vi "Check Instrument Serial Number.vi"(7 "Seq Count":i32, 8 "error in (no error)":errorcluster, 9 "Instrument IDN String (\"\")":string, 11 "Instrument Record":T1) -> (0 "error out":errorcluster)   [LabVIEW 2011]
uses:
  typedefs/Instrument Record.ctl
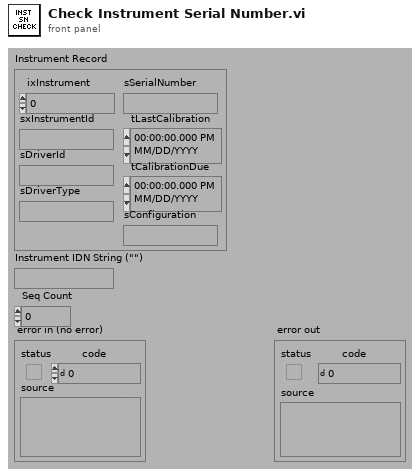
[diagram p1: front panel]
types:
  T1 = typedef "Instrument Record.ctl" = cluster{"ixInstrument":i32, "sxInstrumentId":string, "sDriverId":string, "sDriverType":string, "sSerialNumber":string, "tLastCalibration":timestamp, "tCalibrationDue":timestamp, "sConfiguration":string}
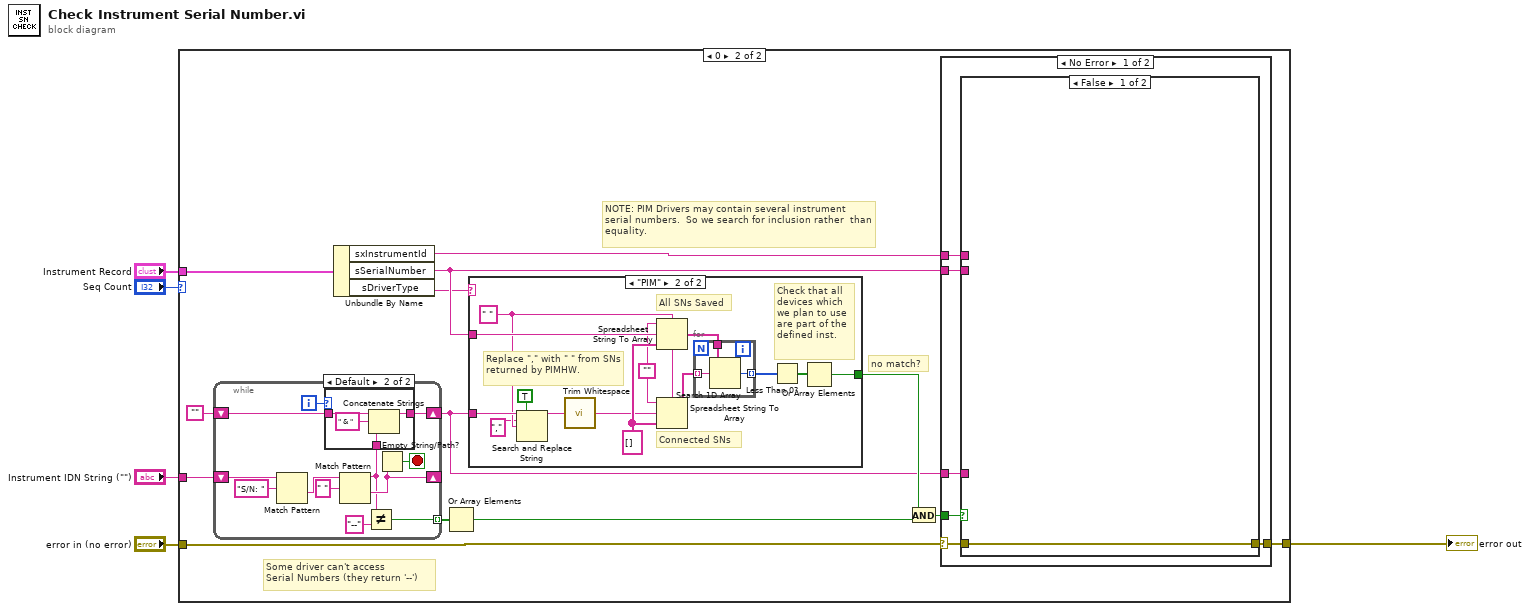
[diagram p0: block diagram]
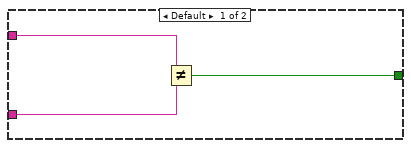
[diagram p3: hidden frame]
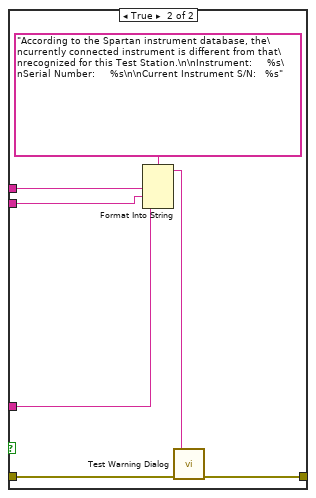
[diagram p5: hidden frame]
diagram:
  n1 = case shown="0" "Seq Count" {
    tunnel: "Instrument Record" -> [_ w18]
    tunnel: [w6 w17] -> w4
    tunnel: "error in (no error)" -> [w6 w16]
    tunnel: "Instrument IDN String (\"\")" -> [_ w13]
    frame Default {
      # "Do not run check if it is not the first time the sequence is run."
    }
    frame 0 {
      # "no match?"
      # "NOTE: PIM Drivers may contain several instrument serial numbers.  So we search for inclusion rather  than equality."
      # "Some driver can't access\nSerial Numbers (they return '--')"
      n2 = while {
        shift-right: [w45] -> _
        shift-left: w13 -> [w50]
        tunnel: [w46] -> w12 mode=indexing
        shift-right: [w41] -> w7
        shift-left: "" -> [w42]
        i -> [w43]
        stop <- w44 stop-if-true
        n3 = Match Pattern(string=w50, regular expression="S/N: ") -> (after substring=w49:string)  [unwired: 4 out]
        n4 = Match Pattern(string=w49, regular expression=" ") -> (before substring=w40:string, after substring=w45:string)  [unwired: 3 out]
        n5 = case shown="Default" w43 {
          tunnel: w42 -> [_ w56]
          tunnel: [w52 w54] -> w41
          tunnel: w40 -> [w52 w55]
          frame 0 {
          }
          frame Default {
            n6 = Concatenate Strings(w56, " & " ("string"), w55) -> (w54:string)
          }
        }
        n7 = Not Equal?(x=w40, y="--" ("x")) -> (x != y?=w46:bool)
        n8 = Empty String/Path?(string/path=w45) -> (empty?=w44:bool)
      }
      n9 = Unbundle By Name(w18) -> ("sxInstrumentId"=w19:string, "sSerialNumber"=w14:string, "sDriverType"=w8:string)
      n10 = Or Array Elements(Boolean array=w12) -> (logical OR=w9:bool)
      n11 = case shown="\"PIM\"" w8 {
        tunnel: w14 -> [w22 w35]
        tunnel: w7 -> [w21 w27]
        tunnel: [w20 w30] -> w10
        frame Default {
          n12 = Not Equal?(x=w22, y=w21) -> (x != y?=w20:bool)
        }
        frame "PIM" {
          w34 = ""
          w36 = string[] []
          w26 = " " ("delimiter (Tab)")
          # "Replace \",\" with \" \" from SNs returned by PIMHW."
          # "Check that all\ndevices which\nwe plan to use\nare part of the\ndefined inst."
          # "Connected SNs"
          # "All SNs Saved"
          n13 = Search and Replace String(replace all?=TRUE ("replace all? (F)"), input string=w27, search string="," ("string"), replace string=w26) -> (result string=w28:string)  [unwired: 1 in, 6 out]
          n14 = call <vilib>:"Trim Whitespace.vi"("string"=w28) -> ("trimmed string"=w23:string)  [unwired: 1 in]
          n15 = Spreadsheet String To Array(delimiter (Tab)=w26, format string=w34, spreadsheet string=w35, array type (2D Dbl)=w36) -> (array=w33:string[])
          n16 = Spreadsheet String To Array(delimiter (Tab)=w26, format string=w34, spreadsheet string=w23, array type (2D Dbl)=w36) -> (array=w32:string[])
          n17 = for {
            tunnel: w33 -> [w39]
            tunnel: w32 -> [w38] mode=indexing
            tunnel: [w37] -> w31 mode=indexing
            n18 = Search 1D Array(1D array=w39, element=w38) -> (index of element=w37:i32)  [unwired: 1 out]
          }
          n19 = Less Than 0?(x=w31) -> (x < 0?=w29:bool[])
          n20 = Or Array Elements(Boolean array=w29) -> (logical OR=w30:bool)
        }
      }
      n21 = And(x=w10, y=w9) -> (x .and. y?=w15:bool)
      n22 = case shown="No Error" w16 {
        selector: w16 -> [w57 w71]
        tunnel: w19 -> [w62 _]
        tunnel: [w61 w71] -> w17
        tunnel: w14 -> [w60 _]
        tunnel: w15 -> [w59 _]
        tunnel: w7 -> [w58 _]
        frame No Error {
          n23 = case shown="False" w59 {
            tunnel: w57 -> [w63 w70]
            tunnel: [w63 w69] -> w61
            tunnel: w62 -> [_ w66]
            tunnel: w60 -> [_ w65]
            tunnel: w58 -> [_ w64]
            frame False {
            }
            frame True {
              n24 = Format Into String(format string="According to the Spartan instrument database, the\ncurrently connected instrument is different from that\nrecognized for this Test Station.\n\nInstrument:     %s\nSerial Number:     %s\n\nCurrent Instrument S/N:   %s", w66, w65, w64) -> (resulting string=w67:string)  [unwired: 2 in, 1 out]
              n25 = call "Test Warning Dialog.vi"("error in (no error)"=w70, "Warning Message"=w67) -> ("error out"=w69:errorcluster)  [unwired: 5 out]
            }
          }
        }
        frame Error {
        }
      }
    }
  }
  "error out" <- w4
